vi "sub_inrange_data.vi"(8 "error in":errorcluster, 10 "limit":dbl, 11 "xy_lidar data":cluster{"x":dbl, "y":dbl}[](array[cluster])) -> (0 "error out":errorcluster, 2 "limit point out":u16, 3 "limit inrange xydata":cluster{"x":dbl, "y":dbl}[](array[cluster]))   [LabVIEW 2019]
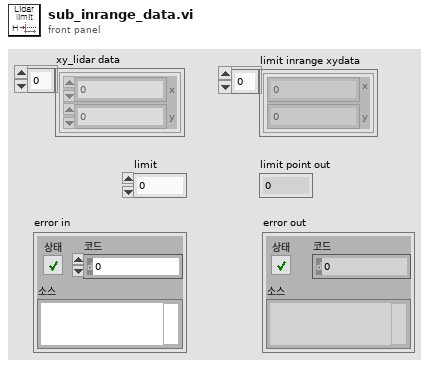
[diagram p1: front panel]
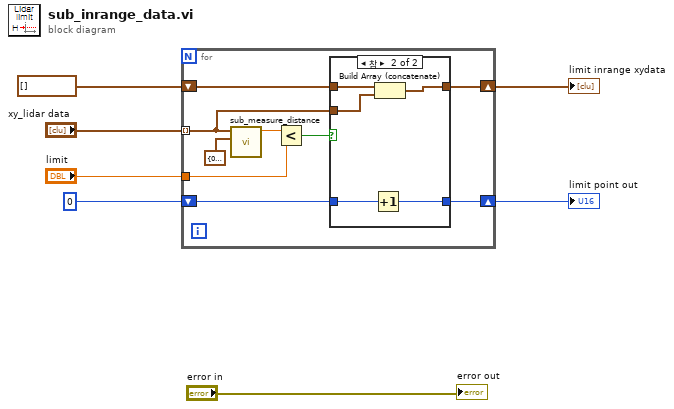
[diagram p0: block diagram]
diagram:
  n1 = for {
    tunnel: "xy_lidar data" -> [w12] mode=indexing
    shift-right: [w11] -> w4
    shift-left: cluster{"x":dbl, "y":dbl}[] [] -> [w10]
    tunnel: "limit" -> [w15]
    shift-right: [w9] -> w7
    shift-left: u16 0 -> [w8]
    n2 = call "sub_measure_distance.vi"("pt 2"=cluster{"x":dbl, "y":dbl} {"x"=0.0, "y"=0.0}, "pt 1"=w12) -> ("distance"=w14:dbl)  [unwired: 9 in]
    n3 = Less?(x=w14, y=w15) -> (x < y?=w13:bool)
    n4 = case shown="참" w13 {
      tunnel: w12 -> [_ w23]
      tunnel: [w18 w22] -> w11
      tunnel: w10 -> [w18 w21]
      tunnel: [w17 w20] -> w9
      tunnel: w8 -> [w17 w19]
      frame False {
      }
      frame True {
        n5 = Increment(x=w19) -> (x+1=w20:u16)
        n6 = Build Array (concatenate)(w21, w23) -> (w22:cluster{"x":dbl, "y":dbl}[])
      }
    }
  }
  "limit point out" <- w7
  "limit inrange xydata" <- w4
  "error out" <- "error in"
